vi "add_to_rio.vi"(4 "to_rio":cluster{"set_speed":dbl, "set_steering":dbl}, 5 "msg in":string) -> (2 "msg out":string)   [LabVIEW 2016]
uses:
  <userlib>/ROS for LabVIEW Software/ROS/MessageBuilding/std_msgs/subs/float64Scalar.vi
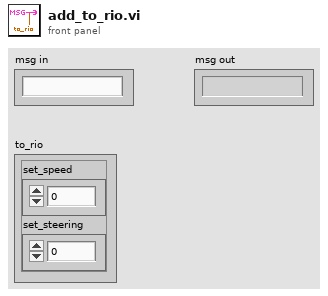
[diagram p1: front panel]
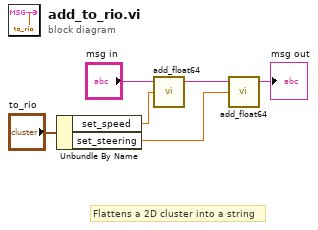
[diagram p0: block diagram]
diagram:
  # "Flattens a 2D cluster into a string"
  n1 = Unbundle By Name("to_rio") -> ("set_speed"=w4:dbl, "set_steering"=w2:dbl)
  n2 = call-poly <userlib>:"add_float64.vi"("Numeric"=w4, "msg in"="msg in") -> ("msg out"=w3:string)  [unwired: 3 in]
  n3 = call-poly <userlib>:"add_float64.vi"("Numeric"=w2, "msg in"=w3) -> ("msg out"=→"msg out":string)  [unwired: 3 in]
